vi "CPP_GetProjectNumber.vi"() -> (3 "ProjectNumber":string)   [LabVIEW 2010]
uses:
  Globals/Preference_global.vi
panel:
  out "RigProjectNumberChannel":string
  out "index of element":i32
  out "Values":string[][](array[string])
  out "Titles":string[](array[string])
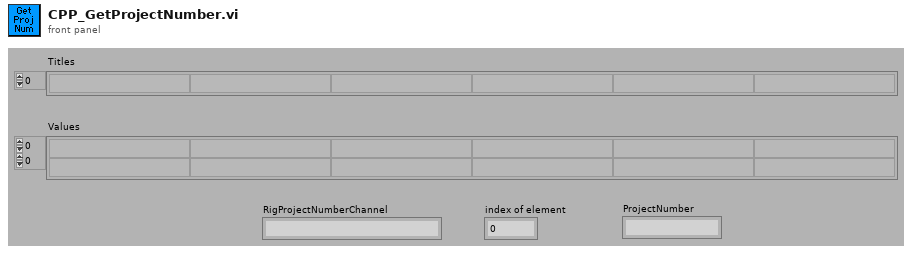
[diagram p1: front panel]
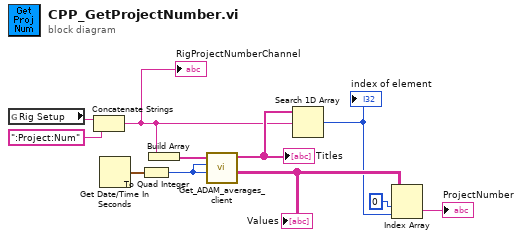
[diagram p0: block diagram]
diagram:
  n1 = global read "Preference_global.vi" "Rig Setup"() -> (w10:string)
  n2 = Concatenate Strings(w10, ":Project:Num" ("element")) -> (w5:string)
  "RigProjectNumberChannel" <- w5
  n3 = Get Date/Time In Seconds() -> (seconds since 1Jan1904=w8:timestamp)
  n4 = To Quad Integer(1:w8) -> (0:w9:i64)
  n5 = Build Array(w5) -> (w6:string[])
  n6 = call "Get_ADAM_averages_client.vi"("End time"=w9, "Start time"=w9, "ADAM Ch Names"=w6) -> ("Values"=w4:string[][], "Titles"=w7:string[])  [unwired: 4 in, 3 out]
  "Titles" <- w7
  "Values" <- w4
  n7 = Search 1D Array(1D array=w7, element=w5) -> (index of element=w3:i32)  [unwired: 1 in]
  "index of element" <- w3
  n8 = Index Array(array=w4, index (row)=0 ("disabled index (row)"), index (col)=w3) -> (element=→"ProjectNumber":string)
